vi "Format Client Request (Numeric).vi"(8 "error in (no error)":errorcluster, 9 "id":i32, 10 "params":refnum<class "JSON Object.lvclass">, 11 "method":string) -> (0 "error out":errorcluster, 2 "Request String":string)   [LabVIEW 2015, in "JSONRPC Server.lvclass"]
uses:
  JSONRPC Server.lvclass
  <vilib>/NI/JSON Support for LabVIEW/JSON Data Classes/JSON Object/JSON Object.lvclass
  <vilib>/NI/JSON Support for LabVIEW/JSON Data Classes/JSON Numeric/New JSON Numeric.vi
  <vilib>/NI/JSON Support for LabVIEW/JSON Data Classes/JSON Object/Insert Key Value Pair (Single).vi
  <vilib>/NI/JSON Support for LabVIEW/JSON Data Classes/JSON Helper/JSON Helper.lvclass
  <vilib>/NI/JSON Support for LabVIEW/JSON Data Classes/JSON Numeric/JSON Numeric.lvclass
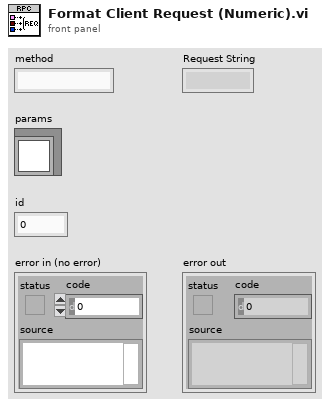
[diagram p1: front panel]
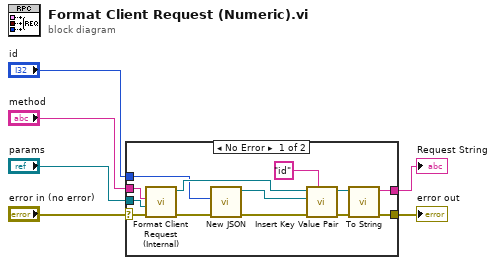
[diagram p0: block diagram]
diagram:
  n1 = case shown="No Error" "error in (no error)" {
    selector: "error in (no error)" -> [w19 w20]
    tunnel: [w18 w20] -> w5
    tunnel: "params" -> [w14 _]
    tunnel: [w17 _] -> w3
    tunnel: "method" -> [w16 _]
    tunnel: "id" -> [w11 _]
    frame No Error {
      n2 = call "Format Client Request (Internal).vi"("error in (no error)"=w19, "params"=w14, "method"=w16) -> ("error out"=w8:errorcluster, "JSON Object out"=w13:refnum<class "JSON Object.lvclass">)  [unwired: 7 in]
      n3 = call-poly <vilib>:"New JSON.vi"("error in (no error)"=w8, "value"=w11) -> ("error out"=w7:errorcluster, "JSON String out"=w10:refnum<class "JSON Numeric.lvclass">)  [unwired: 8 in]
      n4 = call-poly <vilib>:"Insert Key Value Pair.vi"("key"="id" ("Name"), "error in (no error)"=w7, "value"=w10, "JSON Object in"=w13) -> ("error out"=w15:errorcluster, "JSON Object out"=w9:refnum<class "JSON Object.lvclass">)  [unwired: 5 in, 1 out]
      n5 = call-dynamic "To String.vi"("error in (no error)"=w15, "JSON Object in"=w9) -> ("error out"=w18:errorcluster, "String"=w17:string)  [unwired: 8 in]
    }
    frame Error {
    }
  }
  "error out" <- w5
  "Request String" <- w3
